vi "Get XY.vi"(8 "error in (no error)":errorcluster, 10 "Channels":i32[](array[numeric])=[1], 11 "RP Instrument in":refnum<class "RP Instrument.lvclass">) -> (0 "error out":errorcluster, 3 "RP Instrument out":refnum<class "RP Instrument.lvclass">, 4 "Signal":i32[](array[numeric]) format="0x%x (%d)")   [LabVIEW 2019, in "RP Instrument.lvclass"]
uses:
  RP Instrument.lvclass
  RP Status Offsets.ctl
  RP Instrument.lvclass/RP Instrument.ctl
  RP Communicator/RP Communicator.lvclass
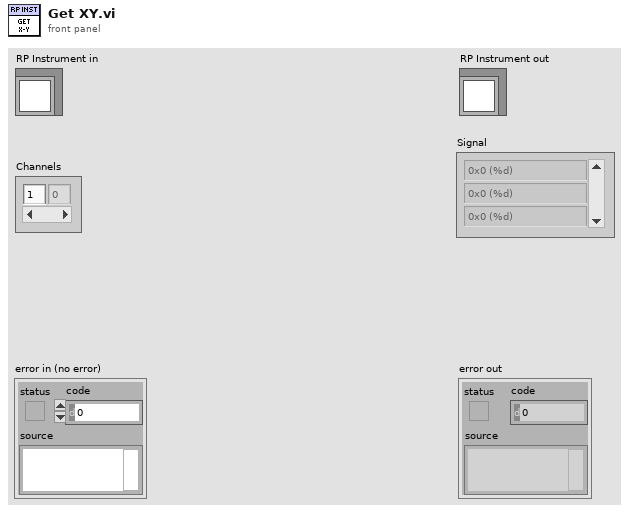
[diagram p1: front panel]
types:
  T1 = typedef "RP Status Offsets.ctl" = u16
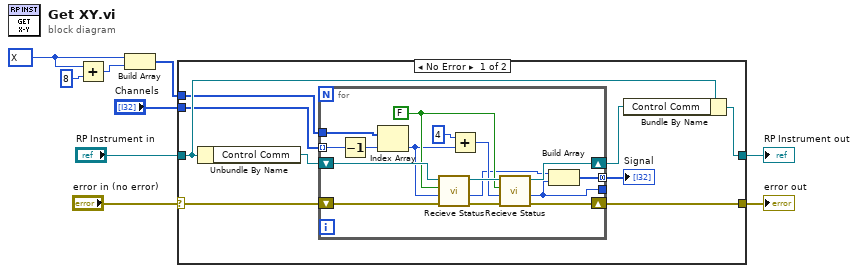
[diagram p0: block diagram]
diagram:
  w2 = T1 16 items=["Writer address"=0, "Record start position"=4, "Trig state and ID"=8, "Phase"=12, "X"=16, "Y"=20, "RxFIFO counter"=24, "TxFIFO counter"=28] ("Status offset")
  n1 = Add(x=w2, y=8) -> (x+y=w3:i32)
  n2 = Build Array(w2, w3) -> (w1:i32[])
  n3 = case shown="No Error" "error in (no error)" {
    selector: "error in (no error)" -> [w17 w36]
    tunnel: [w14 w36] -> w8
    tunnel: [w15 w35] -> w6
    tunnel: "RP Instrument in" -> [w16 w35]
    tunnel: "Channels" -> [w12 _]
    tunnel: w1 -> [w11 _]
    frame No Error {
      n4 = Unbundle By Name(w16) -> ("Control Comm"=w18:refnum<class "RP Communicator.lvclass">)
      n5 = for {
        tunnel: [w20] -> _
        shift-right: [w29] -> w13
        shift-left: w18 -> [w34]
        shift-right: [w31] -> w14
        shift-left: w17 -> [w33]
        tunnel: w12 -> [w26] mode=indexing
        tunnel: w11 -> [w27]
        tunnel: [w19] -> w10 mode=concatenating
        w28 = FALSE ("Read config instead")
        n6 = Decrement(x=w26) -> (x-1=w25:i32)
        n7 = Index Array(array=w27, index=w25) -> (element=w24:i32)
        n8 = call-dynamic "Recieve Status.vi"("error in (no error)"=w33, "Status offset"=w24, "Read config instead"=w28, "RP Communicator in"=w34) -> ("error out"=w32:errorcluster, "Status response"=w21:u32, "RP Communicator out"=w30:refnum<class "RP Communicator.lvclass">)  [unwired: 5 in]
        n9 = Add(x=i64 4, y=w24) -> (x+y=w22:i64)
        n10 = call-dynamic "Recieve Status.vi"("error in (no error)"=w32, "Status offset"=w22, "Read config instead"=w28, "RP Communicator in"=w30) -> ("error out"=w31:errorcluster, "Status response"=w20:u32, "RP Communicator out"=w29:refnum<class "RP Communicator.lvclass">)  [unwired: 5 in]
        n11 = Build Array(w21, w20) -> (w19:u32[])
      }
      "Signal" <- w10
      n12 = Bundle By Name(cluster=w16, "Control Comm"=w13) -> (w15:refnum<class "RP Instrument.lvclass">)
    }
    frame Error {
    }
  }
  "error out" <- w8
  "RP Instrument out" <- w6
